vi "Configure.vi"(8 "error in":errorcluster, 10 "Output Settings":T1={"Voltage (V)"=1.0} {"Voltage (V)" min=-424.2 max=424.2 step=1.0 format="%#.1f"}, 11 "Plugin_Driver in":refnum<class "Plugin_Driver.lvclass">) -> (0 "error out":errorcluster, 3 "Plugin_Driver out":refnum<class "Plugin_Driver.lvclass">)   [LabVIEW 2020, in "Plugin.lvlib" / "Plugin_Driver.lvclass"]
doc: "This VI is a wrapper API for Instrument Driver's Configure API."
uses:
  Plugin_Driver.lvclass
  Drivers/Instrument Driver/Typedefs/Output Settings.ctl
  Drivers/Instrument Driver/Instrument Driver.lvclass
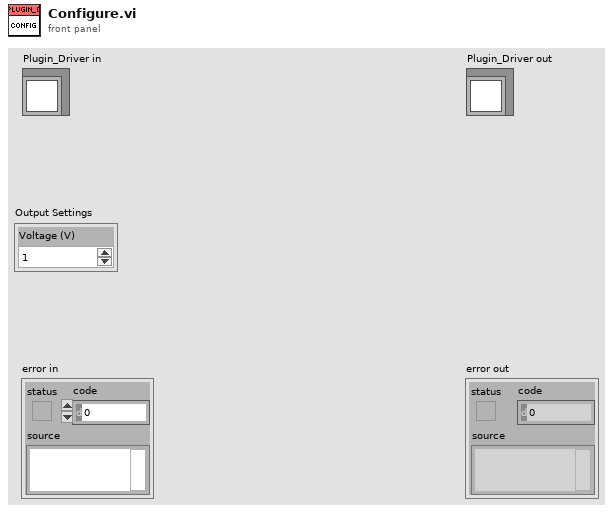
[diagram p1: front panel]
types:
  T1 = typedef "Plugin Instrument Driver.lvlib/Instrument Driver.lvclass/Output Settings.ctl" = cluster{"Voltage (V)":dbl}
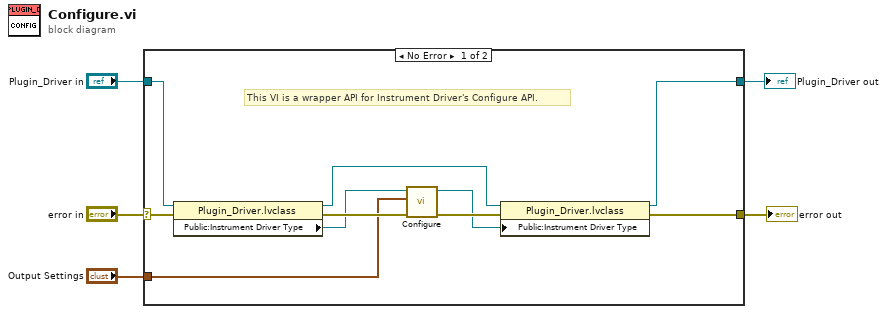
[diagram p0: block diagram]
diagram:
  n1 = case shown="No Error" "error in" {
    selector: "error in" -> [w8 w17]
    tunnel: [w7 w17] -> w4
    tunnel: [w13 w16] -> w2
    tunnel: "Plugin_Driver in" -> [w14 w16]
    tunnel: "Output Settings" -> [w6 _]
    frame No Error {
      # "This VI is a wrapper API for Instrument Driver's Configure API."
      n2 = property class="Plugin_Driver.lvclass"(reference=w14, error in=w8) -> (reference out=w15:refnum<class "Plugin_Driver.lvclass">, error out=w12:errorcluster, "Public:Instrument Driver Type"=w11:refnum<class "Instrument Driver.lvclass">)
      n3 = call-dynamic "Configure.vi"("error in"=w12, "Output Settings"=w6, "Instrument Driver in"=w11) -> ("error out"=w10:errorcluster, "Instrument Driver out"=w9:refnum<class "Instrument Driver.lvclass">)  [unwired: 7 in]
      n4 = property class="Plugin_Driver.lvclass"(reference=w15, error in=w10, "Public:Instrument Driver Type"=w9) -> (reference out=w13:refnum<class "Plugin_Driver.lvclass">, error out=w7:errorcluster)
    }
    frame Error {
    }
  }
  "error out" <- w4
  "Plugin_Driver out" <- w2
